vi "Versioned Write AQT.vi"(10 "data":T1, 11 "Aquitaine paths in":path=path "C:/Users/karth/Documents/Bordeaux Paths/Untitled.aqt") -> (3 "error out":errorcluster)   [LabVIEW 2025]
uses:
  Types/Aquitaine File Data.ctl
  Types/Decision Tree.ctl
  Types/Sequencing Tree Node.ctl
  Types/Single Cmd Info.ctl
  <vilib>/picture/picture.llb/imagedata.ctl
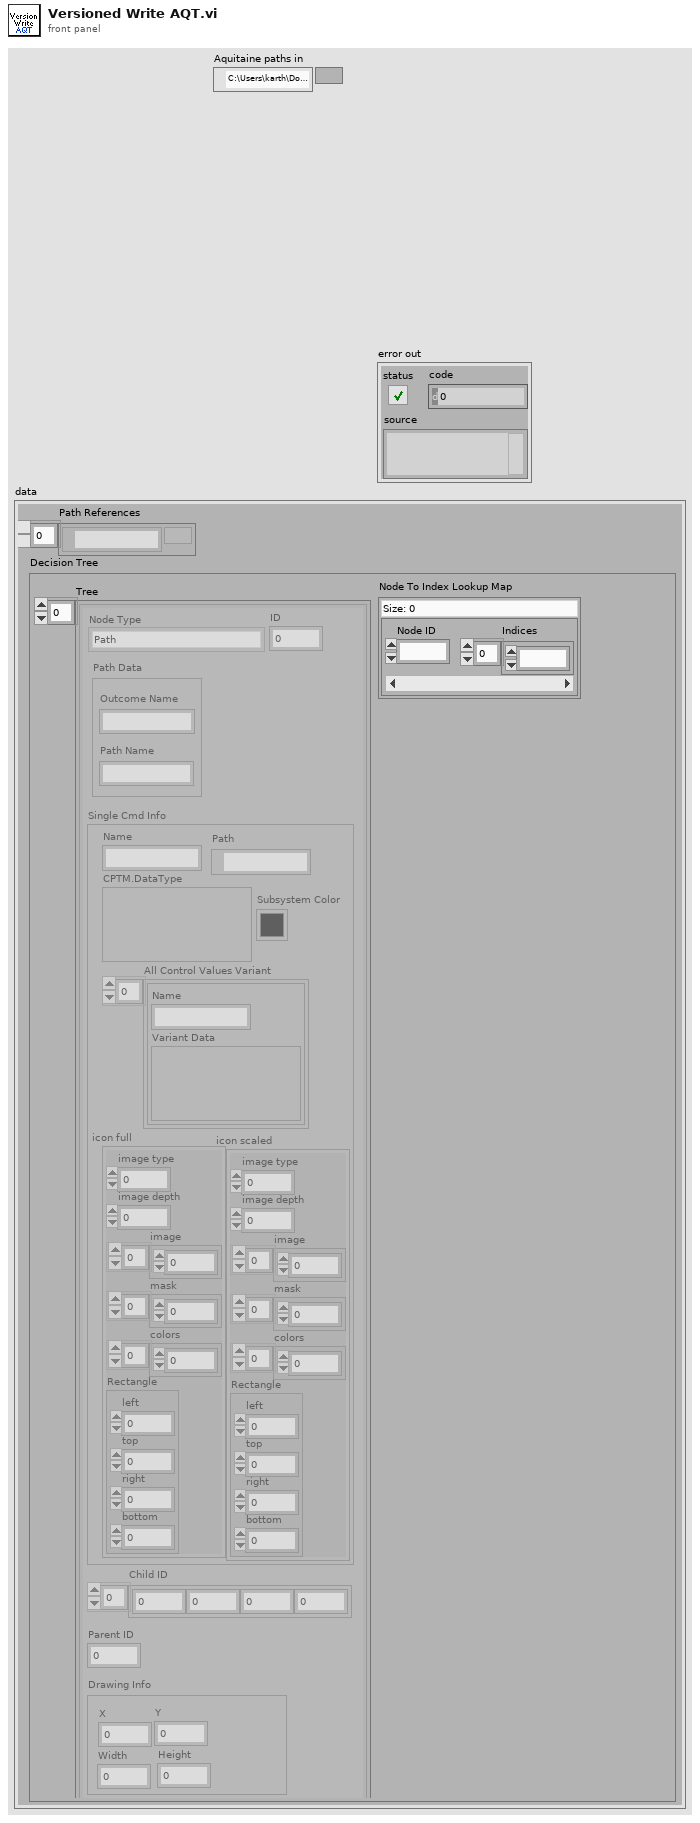
[diagram p1: front panel]
types:
  T1 = typedef "Aquitaine File Data.ctl" = cluster{"Path References":path[], "Decision Tree":T2}
  T2 = typedef "Decision Tree.ctl" = cluster{"Tree":T3[], "Node To Index Lookup Map":map{i16, i16[]}}
  T3 = typedef "Sequencing Tree Node.ctl" = cluster{"Node Type":enum16{"Path", "Command", "Leaf"}, "ID":i16, "Path Data":cluster{"Path Name":string, "Outcome Name":string}, "Single Cmd Info":T4, "Child ID":i32[], "Parent ID":i32, "Drawing Info":cluster{"X":i32, "Y":i32, "Width":i32, "Height":i32}}
  T4 = typedef "Single Cmd Info.ctl" = cluster{"Name":string, "CPTM.DataType":variant, "All Control Values Variant":cluster{"Name":string, "Variant Data":variant}[], "icon full":T5, "icon scaled":T5, "Path":path, "Subsystem Color":u32}
  T5 = typedef "imagedata.ctl" = cluster{"image type":i32, "image depth":i32, "image":u8[], "mask":u8[], "colors":u32[], "Rectangle":cluster{"left":i16, "top":i16, "right":i16, "bottom":i16}}
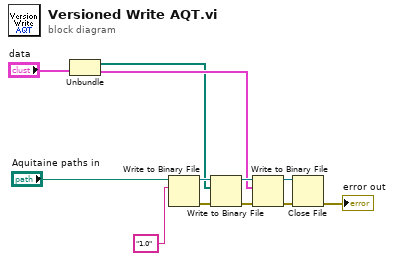
[diagram p0: block diagram]
diagram:
  n1 = Unbundle("data") -> ("Path References"=w5:path[], "Decision Tree"=w6:T2)
  n2 = Write to Binary File(file (use dialog)="Aquitaine paths in", data="1.0") -> (refnum out=w8:refnum<file>, error out=w9:errorcluster)  [unwired: 4 in, 1 out]
  n3 = Write to Binary File(file (use dialog)=w8, data=w5, error in=w9) -> (refnum out=w10:refnum<file>, error out=w11:errorcluster)  [unwired: 3 in, 1 out]
  n4 = Write to Binary File(file (use dialog)=w10, data=w6, error in=w11) -> (refnum out=w2:refnum<file>, error out=w1:errorcluster)  [unwired: 3 in, 1 out]
  n5 = Close File(refnum=w2, error in=w1) -> (error out=→"error out":errorcluster)  [unwired: 1 out]
